vi "Generate Icon Text.vi"(8 "error in (no error)":errorcluster, 11 "Getter Generator in":refnum<class "Getter Generator.lvclass">) -> (0 "error out":errorcluster, 3 "Getter Generator out":refnum<class "Getter Generator.lvclass">)   [LabVIEW 2020, in "Method Generation.lvlib" / "Getter Generator.lvclass"]
uses:
  Getter Generator.lvclass
  Support/Support.lvlib
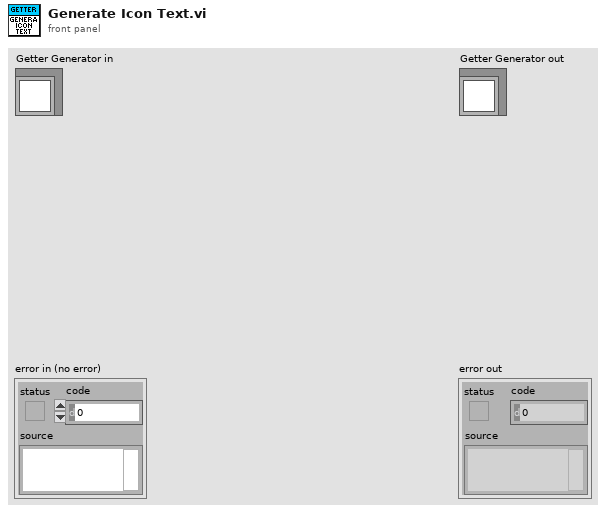
[diagram p1: front panel]
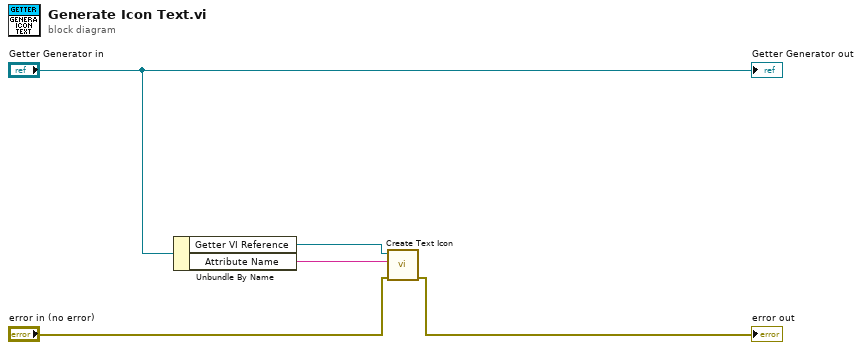
[diagram p0: block diagram]
diagram:
  n1 = Unbundle By Name("Getter Generator in") -> ("Getter VI Reference"=w3:refnum<vi>, "Attribute Name"=w4:string)
  n2 = call "Create Text Icon.vi"("error in (no error)"="error in (no error)", "Icon Text String"=w4, "VI in"=w3) -> ("error out"=→"error out":errorcluster)  [unwired: 7 in, 1 out]
  "Getter Generator out" <- "Getter Generator in"
